vi "Bounding-box angles.vi"(6 "Camera angle offset (rad)":dbl, 8 "Camera Info":T1, 11 "Bounding Box":T2) -> (3 "Bounding box (radians)":T2)   [LabVIEW 2012]
uses:
  CameraResolutionInfo.ctl
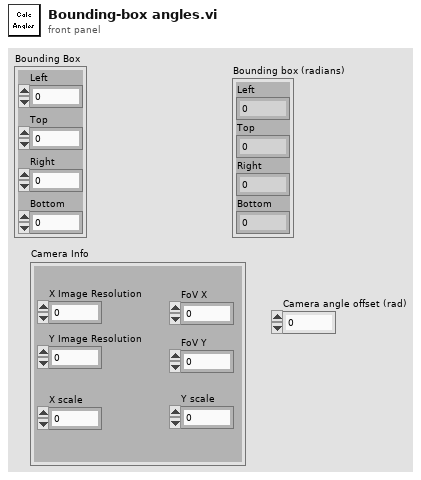
[diagram p1: front panel]
types:
  T1 = typedef "CameraResolutionInfo.ctl" = cluster{"X Image Resolution":i32, "Y Image Resolution":i32, "FoV X":dbl, "FoV Y":dbl, "X scale":dbl, "Y scale":dbl}
  T2 = cluster{"Left":dbl, "Top":dbl, "Right":dbl, "Bottom":dbl}
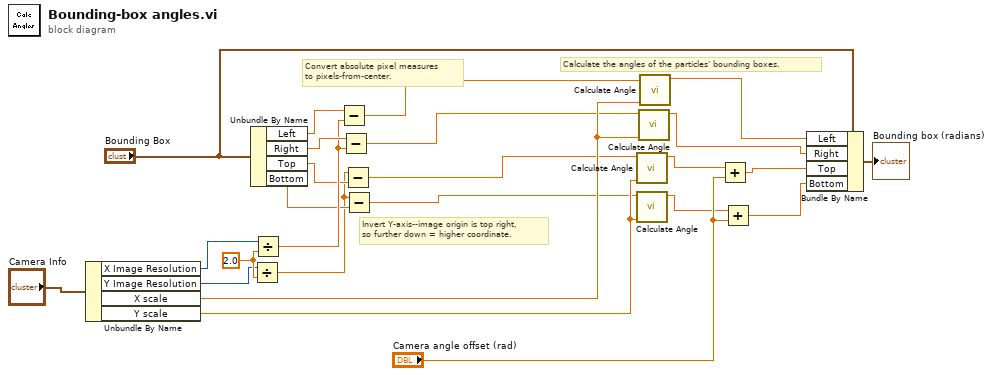
[diagram p0: block diagram]
diagram:
  w13 = 2.0
  # "Invert Y-axis--image origin is top right,\nso further down = higher coordinate."
  # "Convert absolute pixel measures\nto pixels-from-center."
  # "Calculate the angles of the particles' bounding boxes."
  n1 = Unbundle By Name("Camera Info") -> ("X Image Resolution"=w12:i32, "Y Image Resolution"=w11:i32, "X scale"=w20:dbl, "Y scale"=w19:dbl)
  n2 = Unbundle By Name("Bounding Box") -> ("Left"=w10:dbl, "Right"=w9:dbl, "Top"=w5:dbl, "Bottom"=w4:dbl)
  n3 = Divide(x=w11, y=w13) -> (x/y=w3:dbl)
  n4 = Divide(x=w12, y=w13) -> (x/y=w6:dbl)
  n5 = Subtract(x=w10, y=w6) -> (x-y=w8:dbl)
  n6 = Subtract(x=w9, y=w6) -> (x-y=w7:dbl)
  n7 = Subtract(x=w3, y=w5) -> (x-y=w2:dbl)
  n8 = Subtract(x=w3, y=w4) -> (x-y=w1:dbl)
  n9 = call "Calculate Angle.vi"("Pixel Divisor"=w19, "Pixel In"=w2) -> ("Angle Out (Rad)"=w18:dbl)  [unwired: 9 in]
  n10 = call "Calculate Angle.vi"("Pixel Divisor"=w19, "Pixel In"=w1) -> ("Angle Out (Rad)"=w14:dbl)  [unwired: 9 in]
  n11 = call "Calculate Angle.vi"("Pixel Divisor"=w20, "Pixel In"=w7) -> ("Angle Out (Rad)"=w23:dbl)  [unwired: 9 in]
  n12 = call "Calculate Angle.vi"("Pixel Divisor"=w20, "Pixel In"=w8) -> ("Angle Out (Rad)"=w24:dbl)  [unwired: 9 in]
  n13 = Add(x=w18, y="Camera angle offset (rad)") -> (x+y=w17:dbl)
  n14 = Add(x=w14, y="Camera angle offset (rad)") -> (x+y=w16:dbl)
  n15 = Bundle By Name(cluster="Bounding Box", "Left"=w24, "Right"=w23, "Top"=w17, "Bottom"=w16) -> (→"Bounding box (radians)":T2)
